vi "SelectMenu.vi"(0 "XRef":T13, 1 "Tag":T9, 2 "Point":T11, 3 "Click Type":T10, 4 "State In":T1 {"BlockNodeState"."Draw Style" items=["FunctionBlock", "ExpressVI", "Variable", "Elemental I/O", "32x32 Icon", "FunctionBlockCompact"]; "BlockNodeState"."Terminal Data"."Terminal Flags" format="%.0b"}) -> (14 "Reply":T8, 16 "State Out":T1 {"BlockNodeState"."Draw Style" items=["FunctionBlock", "ExpressVI", "Variable", "Elemental I/O", "32x32 Icon", "FunctionBlockCompact"]; "BlockNodeState"."Terminal Data"."Terminal Flags" format="%.0b"})   [LabVIEW 2020, in "Get DDT Properties.lvlib" / "Get DDT Properties.xnode"]
uses:
  <vilib>/express/express signal manip/GetorSetDDTAttributes/Get DDT Attributes/Get DDT Properties.xnode
  <vilib>/XNodeSupport/XNodeXNodeRef.ctl
  <vilib>/XNodeSupport/XNodeString.ctl
  <vilib>/XNodeSupport/XNodePoint.ctl
  <vilib>/XNodeSupport/XNodeInt.ctl
  <vilib>/XNodeSupport/XNodeClickTypes.ctl
  <vilib>/express/express signal manip/GetorSetDDTAttributes/Get DDT Attributes/State.ctl
  <vilib>/BlockNodeSupport/BlockNodeState.ctl
  <vilib>/BlockNodeSupport/TerminalData.ctl
  <vilib>/picture/picture.llb/imagedata.ctl
  <vilib>/express/express signal manip/GetorSetDDTAttributes/Shared VIs/Attributes data.ctl
  <vilib>/express/express signal manip/GetorSetDDTAttributes/Shared VIs/Input.ctl
  <vilib>/express/express signal manip/GetorSetDDTAttributes/Shared VIs/Attributes name.ctl
  <vilib>/XNodeSupport/XNodeStringArray.ctl
  <vilib>/XNodeSupport/NI_XNodeSupport.lvlib
  <vilib>/express/express signal manip/GetorSetDDTAttributes/Get DDT Attributes/Get DDT Properties.lvlib
  <vilib>/express/express signal manip/GetorSetDDTAttributes/Shared VIs/GetSetShared.lvlib
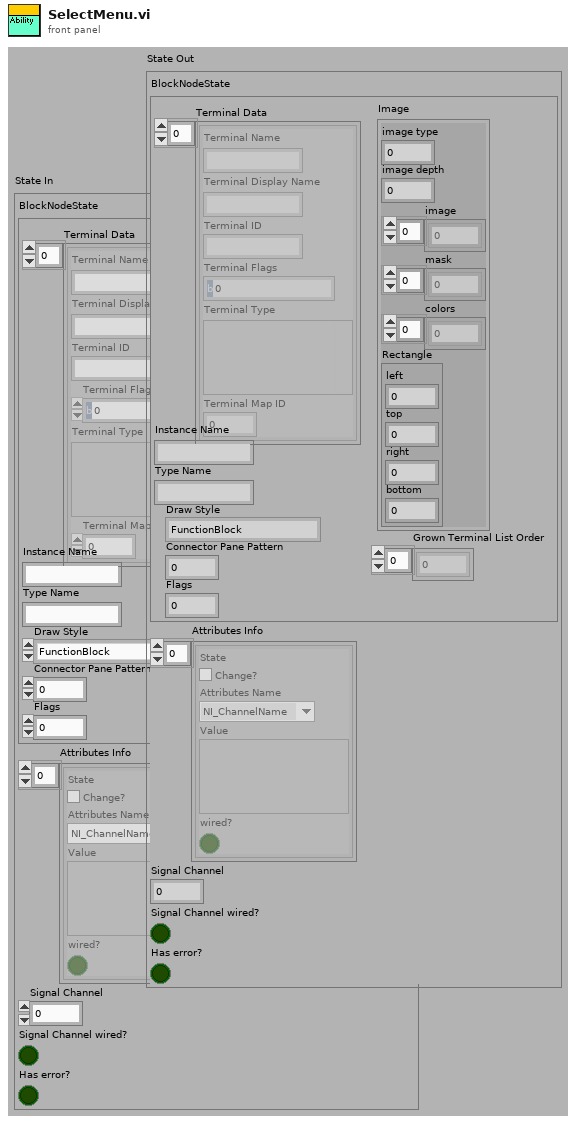
[diagram p1: front panel]
types:
  T1 = typedef "Get DDT Properties.lvlib/Get DDT Properties.xnode/State.ctl" = cluster{"BlockNodeState":T2, "Attributes Info":T5[], "Signal Channel":u32, "Signal Channel wired?":bool, "Has error?":bool}
  T2 = typedef "BlockNodeState.ctl" = cluster{"Terminal Data":T3[], "Instance Name":string, "Type Name":string, "Draw Style":i32, "Connector Pane Pattern":i32, "Flags":i32, "Grown Terminal List Order":i32[], "Image":T4}
  T3 = typedef "TerminalData.ctl" = cluster{"Terminal Name":string, "Terminal Display Name":string, "Terminal ID":string, "Terminal Flags":i32, "Terminal Type":variant, "Terminal Map ID":i32}
  T4 = typedef "imagedata.ctl" = cluster{"image type":i32, "image depth":i32, "image":u8[], "mask":u8[], "colors":u32[], "Rectangle":cluster{"left":i16, "top":i16, "right":i16, "bottom":i16}}
  T5 = typedef "GetSetShared.lvlib/Attributes data.ctl" = cluster{"State":T6, "Attributes Name":T7, "Value":variant, "wired?":bool}
  T6 = typedef "GetSetShared.lvlib/Input.ctl" = bool
  T7 = typedef "GetSetShared.lvlib/Attributes name.ctl" = enum16{"NI_ChannelName", "NI_ExpIsRelativeTime", "NI_ExpTimeStamp", "NI_ExpStartTimeStamp", "NI_ExpXDimension", "NI_UnitDescription"}
  T8 = typedef "NI_XNodeSupport.lvlib/XNodeStringArray.ctl" = T9[]
  T9 = typedef "NI_XNodeSupport.lvlib/XNodeString.ctl" = string
  T10 = typedef "NI_XNodeSupport.lvlib/XNodeClickTypes.ctl" = enum32{"Operate Click", "Popup Click"}
  T11 = typedef "NI_XNodeSupport.lvlib/XNodePoint.ctl" = cluster{"H":T12, "V":T12}
  T12 = typedef "NI_XNodeSupport.lvlib/XNodeInt.ctl" = i32
  T13 = typedef "NI_XNodeSupport.lvlib/XNodeXNodeRef.ctl" = refnum<vi>
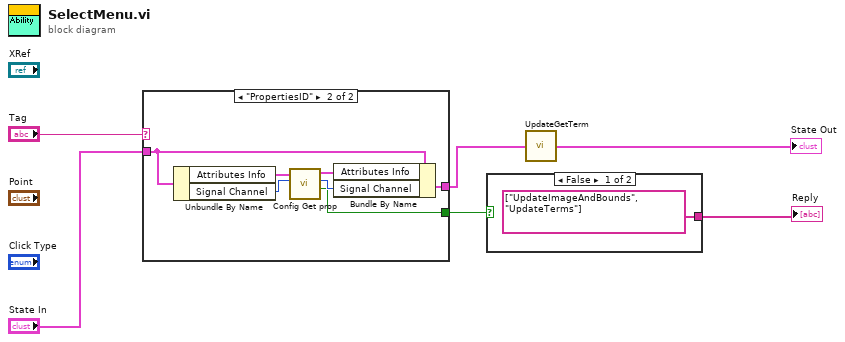
[diagram p0: block diagram]
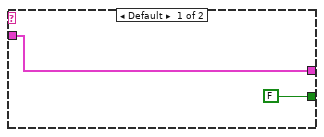
[diagram p3: hidden frame]
diagram:
  n1 = case shown="\"PropertiesID\"" "Tag" {
    tunnel: "State In" -> [w7 w15]
    tunnel: [FALSE ("Cancelled?") w9] -> w6
    tunnel: [w7 w14] -> w2
    frame Default {
    }
    frame "PropertiesID" {
      n2 = Unbundle By Name(w15) -> ("Attributes Info"=w13:T5[], "Signal Channel"=w12:u32)
      n3 = call <vilib>:"Config Get prop.vi"("Signal Channel"=w12, "Attributes in"=w13) -> ("Cancelled?"=w9:bool, "Channel out"=w11:u32, "Attributes out"=w10:T5[])  [unwired: 7 out]
      n4 = Bundle By Name(cluster=w15, "Attributes Info"=w10, "Signal Channel"=w11) -> (w14:T1)
    }
  }
  n5 = case shown="False" w6 {
    tunnel: [T8 ["UpdateImageAndBounds", "UpdateTerms"] ("Reply") _] -> w3
    frame False {
    }
    frame True {
    }
  }
  "Reply" <- w3
  n6 = call <vilib>:"UpdateGetTerm.vi"("State In"=w2) -> ("State Out"=→"State Out":T1)
